vi "3D-CollectProgramName.vi"(11 "路径":path) -> (3 "文件夹名":string[](array[string]))   [LabVIEW 2015]
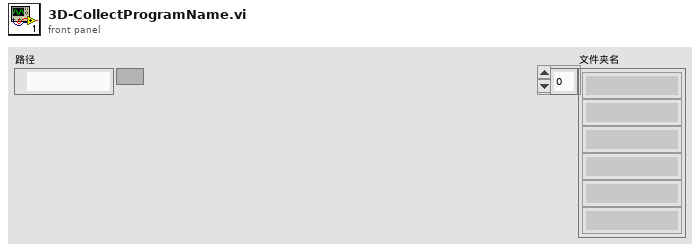
[diagram p1: front panel]
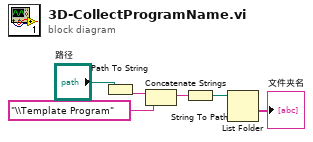
[diagram p0: block diagram]
diagram:
  n1 = Path To String(path="路径") -> (string=w6:string)
  n2 = Concatenate Strings(w6, "\\Template Program" ("字符串")) -> (w4:string)
  n3 = String To Path(string=w4) -> (path=w3:path)
  n4 = List Folder(path=w3) -> (folder names=→"文件夹名":string[])  [unwired: 3 in, 3 out]
